vi "Mindsensors RTC-NX Config.vi"(10 "Node Data":T1, 11 "NXT":T2) -> ()   [LabVIEW 2010]
uses:
  <vilib>/NXT/Subs/LVHSConnector.ctl
  Datatypes/Node.ctl
  UI Controls/PlugInControls/Pluginbackground.ctl
  <vilib>/Utility/miscctls.llb/LVPointTypeDef.ctl
  ConvertNodeAddrSensor.vi
panel:
  out "Date":string
  out "Time":string
  in  "Clock Reading:":string
  out "?":u8 format="%x"
  out "?":dbl format="%#.2g"
  out "number":i8
  in  "Device Address":string
  in  "NXT Port":string
  in  "Name":string
  out "Headline":string="Type (auto populated)"
  in  "Sensor Parameters":string
  in  "Instance Specific Data":cluster{"Example Data":dbl}
  in  "Reset":bool
  in  "Save":bool
  in  "Stop":bool
  out "Background":T3=TRUE
  # "<- No controls below this line"
  # "Common controls such as Buttons, Rings, Sliders, Graphs, Decorations, etc can be found in the <labview>\\Targets\\NI\\NXT\\NXT Toolkit\\Schematic Editor\\UI Controls\\Plugin Controls\\ folder. Use these controls when possible to ensure a consistent look and feel with LabVIEW Education Edition."
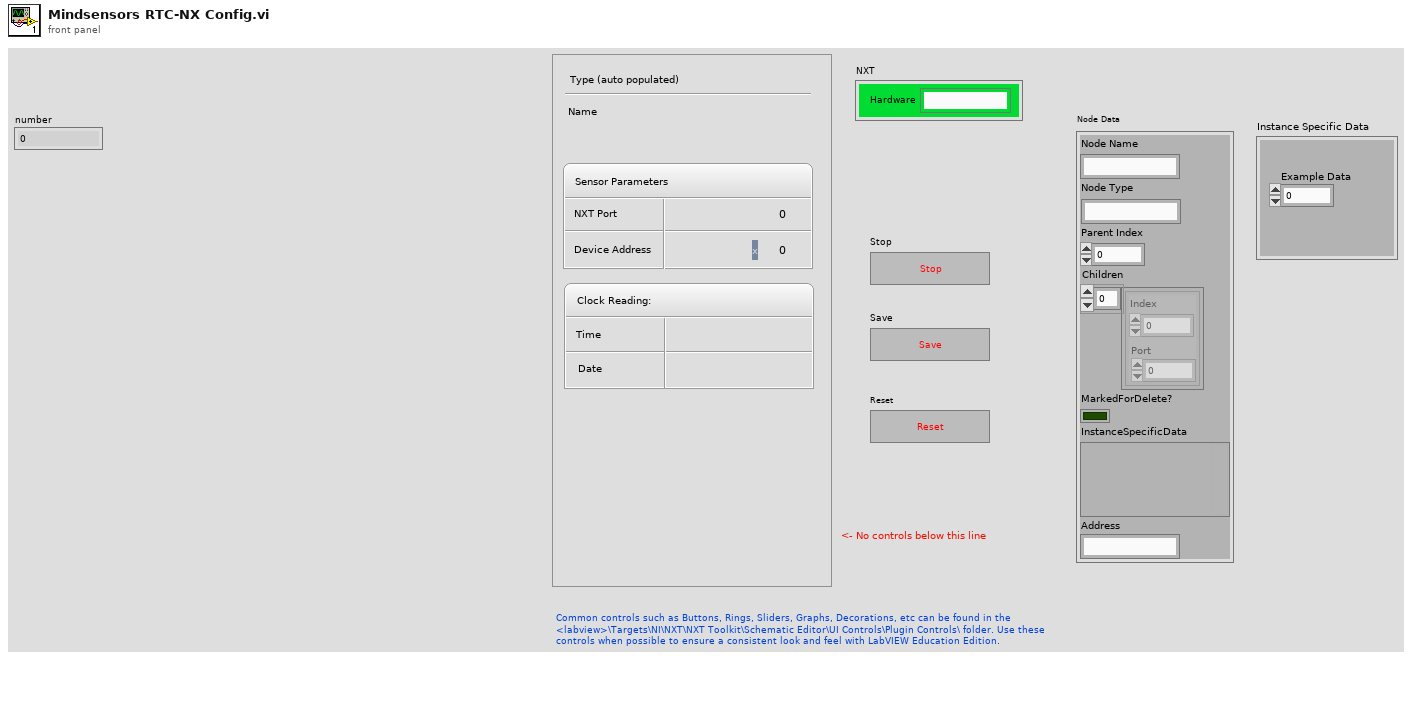
[diagram p1: front panel]
types:
  T1 = typedef "Node.ctl" = cluster{"Node Name":string, "Node Type":string, "Parent Index":i16, "Children":cluster{"Index":u16, "Port":u16}[], "MarkedForDelete?":bool, "InstanceSpecificData":variant, "Address":string}
  T2 = typedef "LVHSConnector.ctl" = cluster{"Hardware":string, "Flattened String":string}
  T3 = typedef "Pluginbackground.ctl" = bool
  T4 = typedef "LVPointTypeDef.ctl" = cluster{"Horizontal":i16, "Vertical":i16}
  T5 = enum8{"Enabled", "Disabled", "Disabled and Grayed Out"}
  T6 = typedef "NXT_InputPort.ctl" = u8
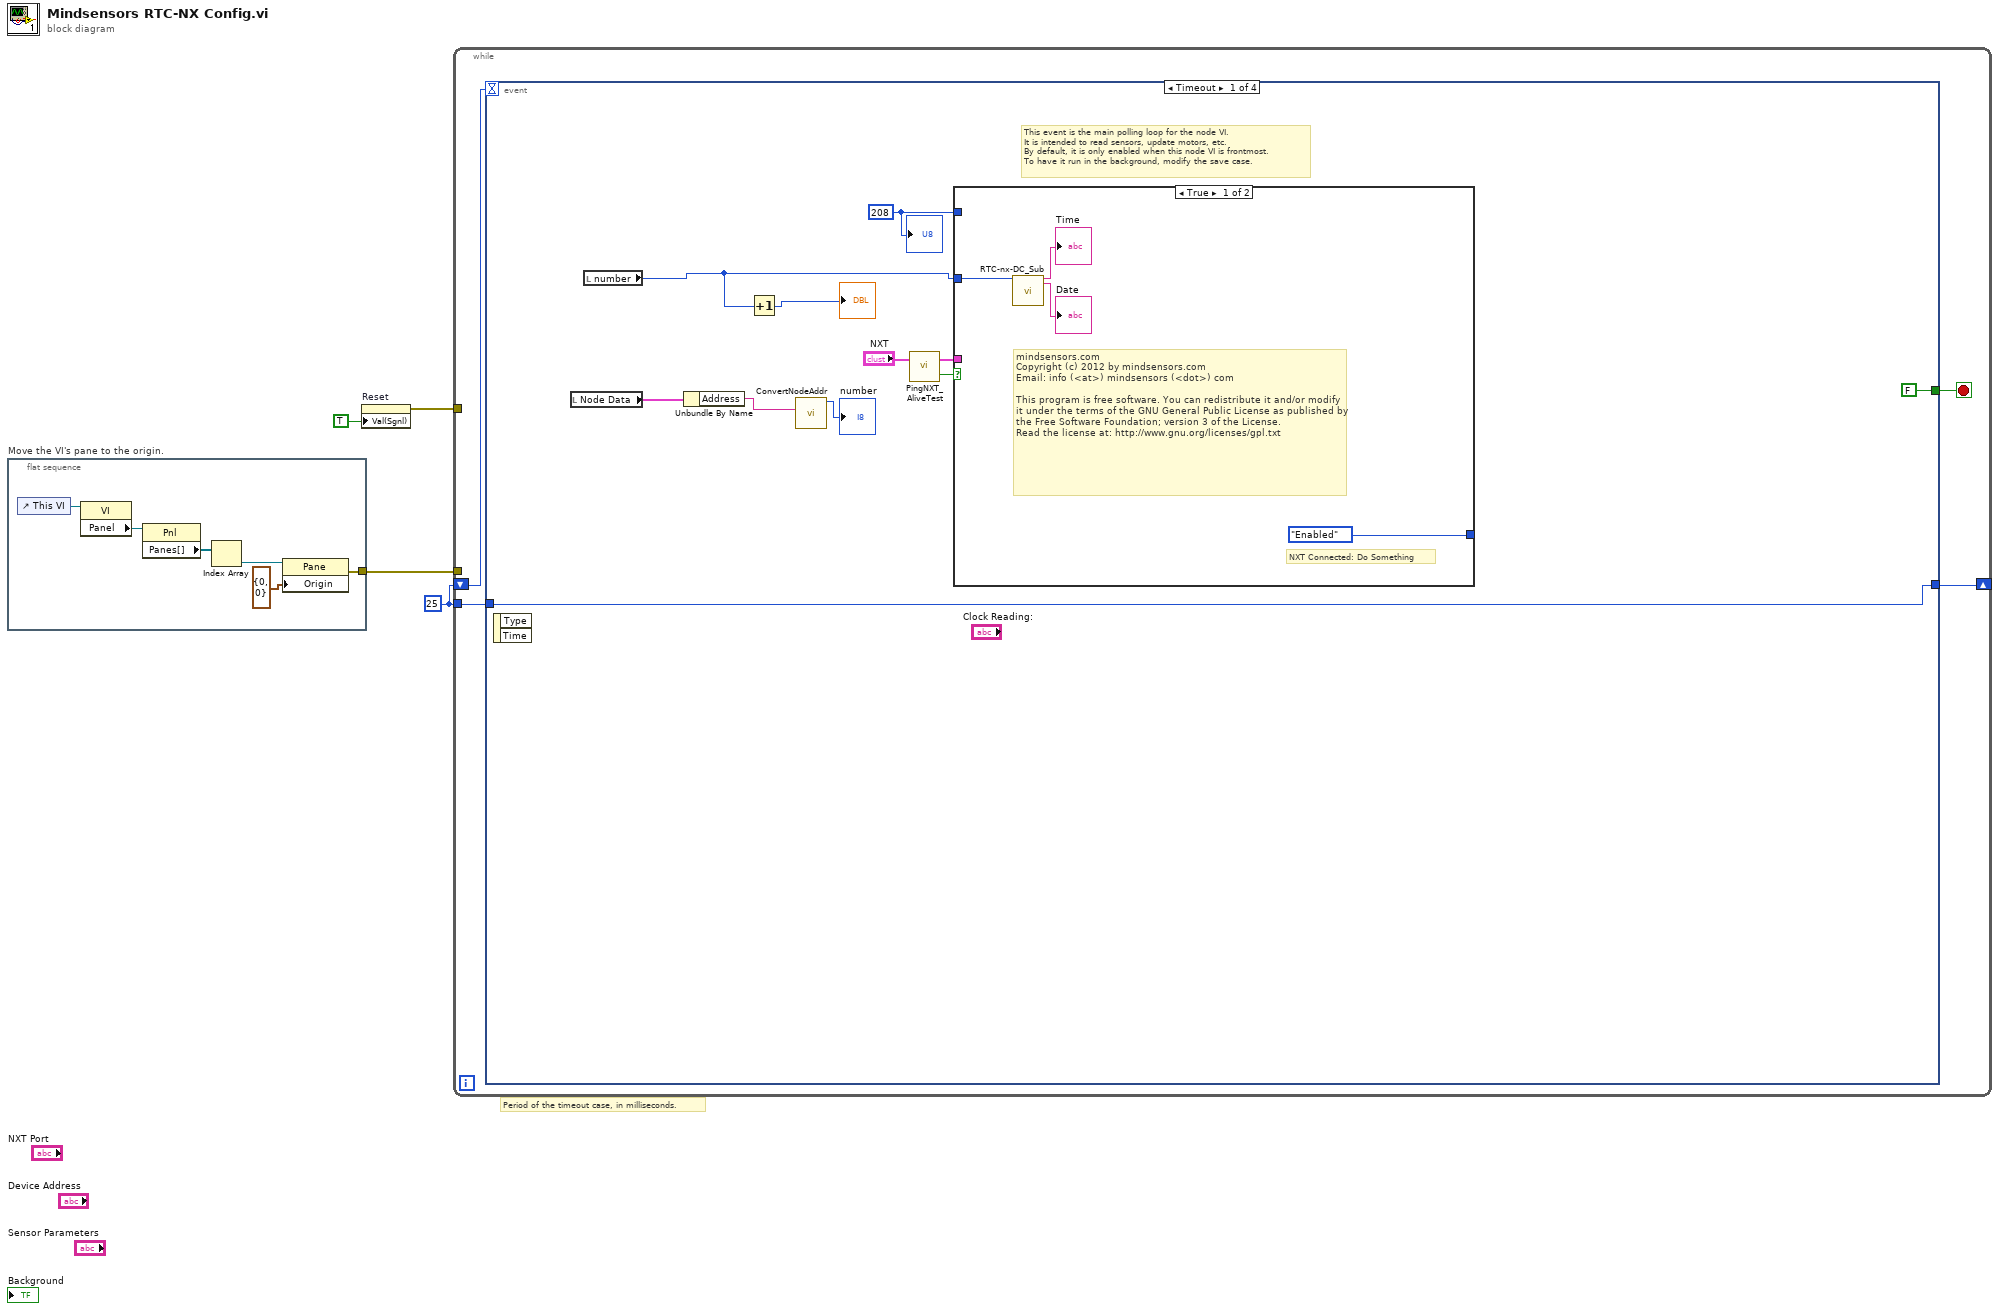
[diagram p0: block diagram]
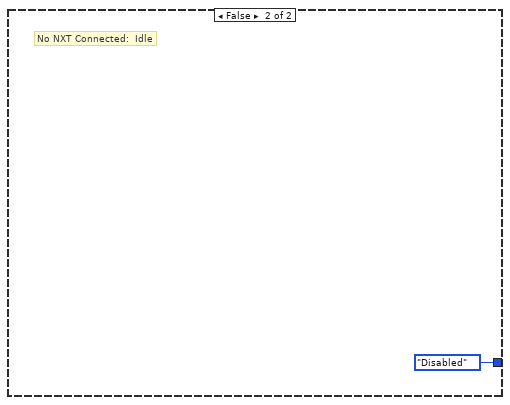
[diagram p2: hidden frame]
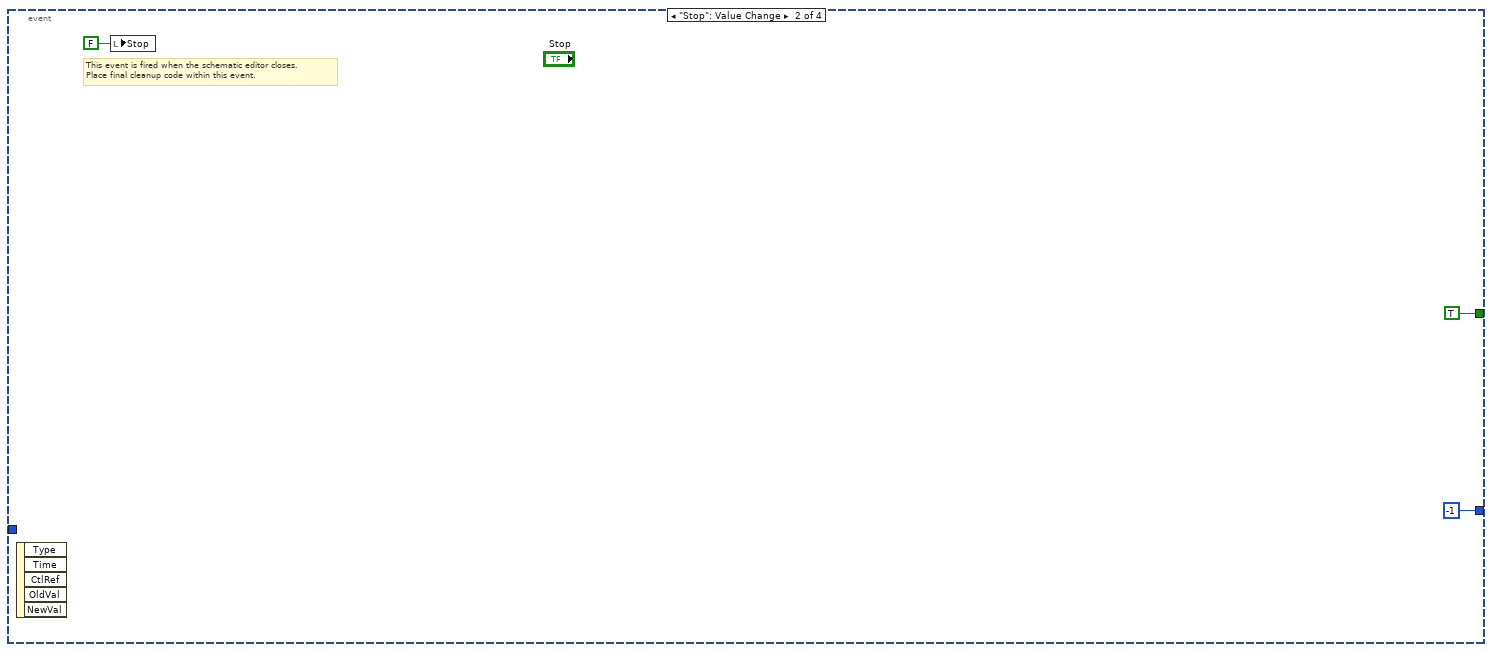
[diagram p3: hidden frame]
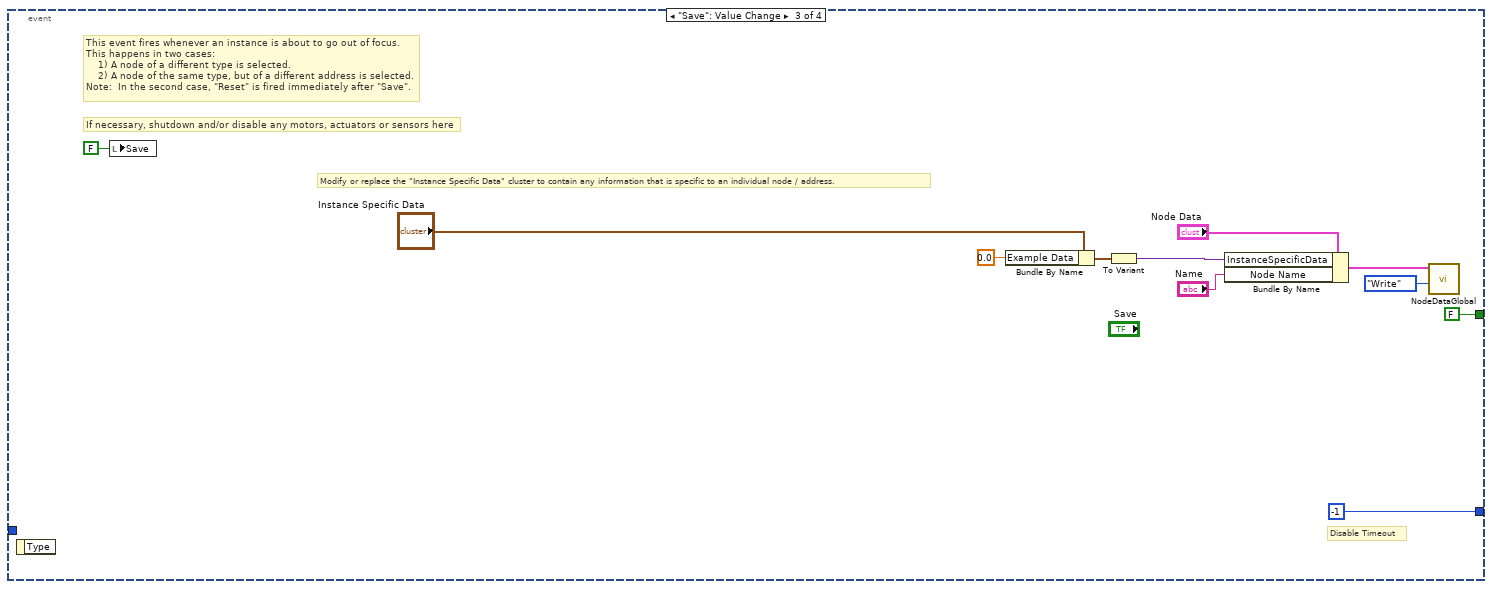
[diagram p4: hidden frame]
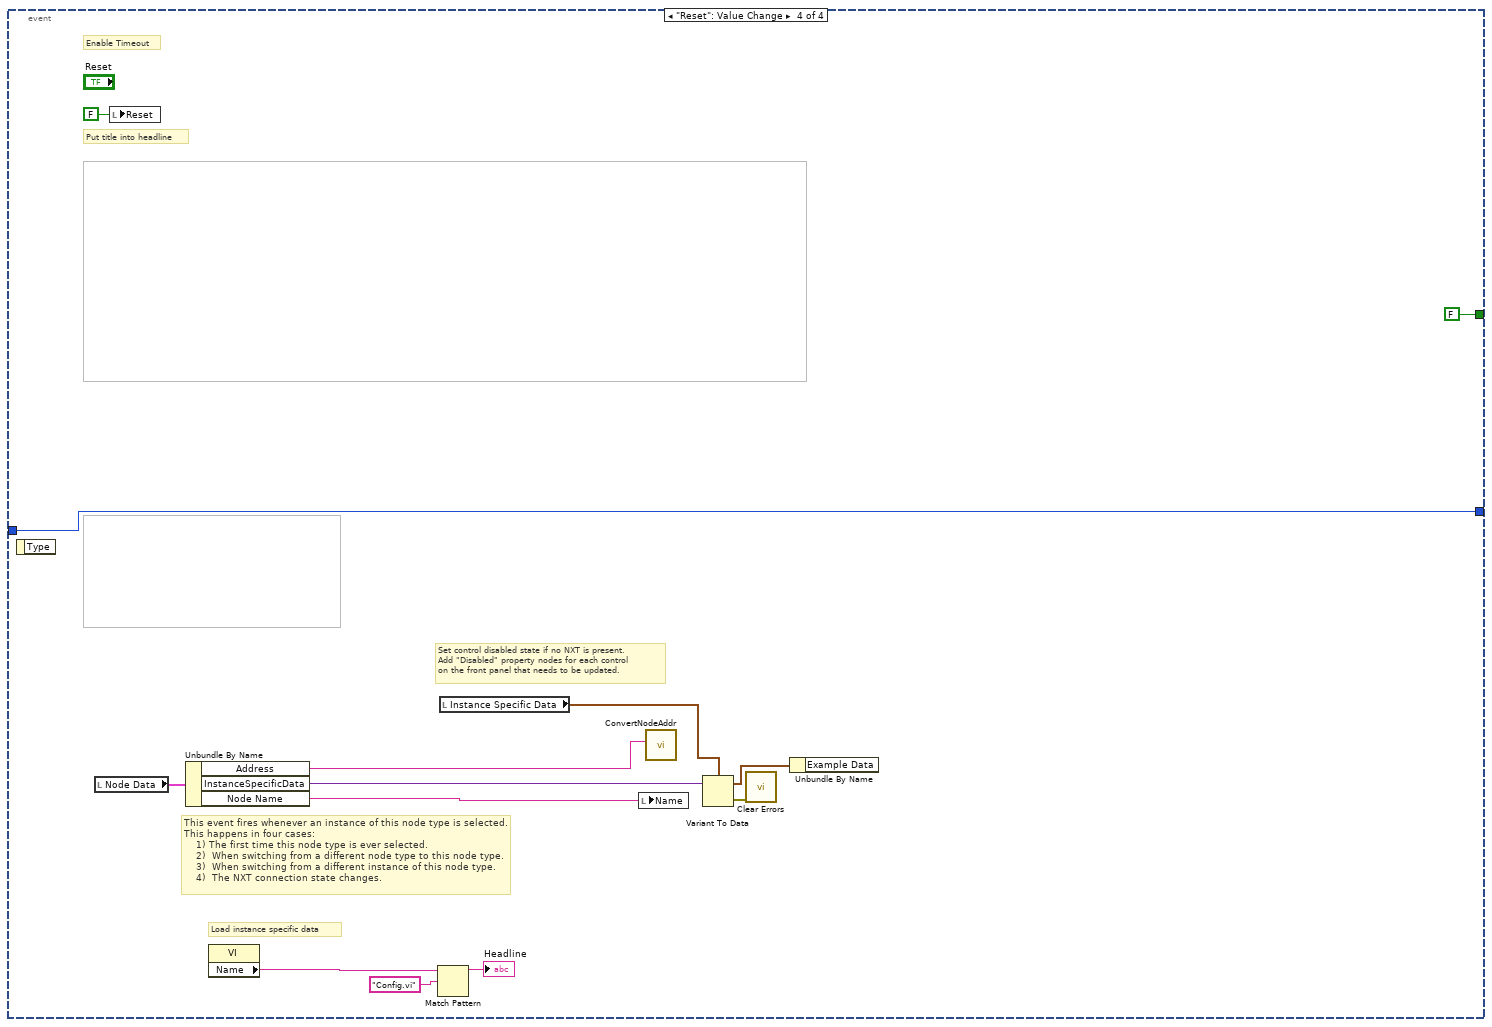
[diagram p5: hidden frame]
diagram:
  w2 = 25
  # "Period of the timeout case, in milliseconds."
  n1 = flat-sequence "Move the VI's pane to the origin." {
    tunnel: [w5] -> w1
    frame #0 {
      n2 = control-ref of="This VI"() -> (w6:refnum<vi>)
      n3 = property class="VI"(reference=w6) -> ("Panel"=w7:refnum<vi>)  [unwired: 1 in, 2 out]
      n4 = property class="Pnl"(reference=w7) -> ("Panes[]"=w8:refnum<vi>[])  [unwired: 1 in, 2 out]
      n5 = Index Array(array=w8) -> (element=w9:refnum<vi>)  [unwired: 1 in]
      n6 = property class="Pane"(reference=w9, "Origin"=T4 {"Horizontal"=0, "Vertical"=0}) -> (error out=w5:errorcluster)  [unwired: 1 in, 1 out]
    }
  }
  n7 = property on="Reset" class="Bool (strict)"("Val(Sgnl)"=TRUE ("Value (Signaling)")) -> (error out=w3:errorcluster)  [unwired: 2 in, 1 out]
  n8 = while {
    tunnel: w3 -> [_]
    shift-right: [w12] -> _
    shift-left: w2 -> [w13]
    tunnel: w2 -> [w11]
    tunnel: w1 -> [_]
    stop <- w14 stop-if-true
    n9 = event shown="[0] Timeout" {
      selector: _ -> [_ _ _ _]
      dyn-events: _ -> [_ _ _ _]
      timeout: w13 -> [_ _ _ _]
      tunnel: [FALSE TRUE FALSE FALSE] -> w14
      tunnel: [w24 -1 -1 w53] -> w12
      tunnel: w11 -> [w24 _ _ w53]
      event Timeout {
        w19 = 208 ("Registry Address")
        # "This event is the main polling loop for the node VI.\nIt is intended to read sensors, update motors, etc.\nBy default, it is only enabled when this node VI is frontmost.\nTo have it run in the background, modify the save case."
        n10 = event-data() -> ()  [unwired: 1 in, 2 out]
        n11 = local read "Node Data"() -> (w22:T1)
        n12 = local read "number"() -> (w16:i8)
        n13 = Unbundle By Name(w22) -> ("Address"=w18:string)
        n14 = Increment(x=w16) -> (x+1=→"?":i8)
        n15 = call-poly "ConvertNodeAddr.vi"("Sensor Port"=w18) -> ("NXT Port"=→"number":T6)  [unwired: 6 in, 4 out]
        n16 = call <vilib>:"PingNXT_AliveTest.vi"("NXT"="NXT") -> ("connected?"=w21:bool, "NXT"=w20:T2)  [unwired: 1 in]
        n17 = case shown="True" w21 {
          tunnel: [T5."Enabled" ("Disabled") T5."Disabled" ("Disabled")] -> _
          tunnel: w20 -> [_ _]
          tunnel: w16 -> [w28 _]
          tunnel: w19 -> [_ _]
          frame True {
            # "mindsensors.com\nCopyright (c) 2012 by mindsensors.com\nEmail: info (<at>) mindsensors (<dot>) com\n\nThis program is free software. You can redistribute it and/or modify\nit under the terms of the GNU General Public License as published by\nthe Free Software Foundation; version 3 of the License.\nRead the license at: http://www.gnu.org/licenses/gpl.txt"
            # "NXT Connected: Do Something"
            n18 = call <vilib>:"RTC-nx-DC_Sub.vi"("Input Port (Port 1)"=w28) -> ("time string"=→"Time":string, "date string"=→"Date":string)  [unwired: 10 in, 7 out]
          }
          frame False {
            # "No NXT Connected:  Idle"
          }
        }
        "?" <- w19
      }
      event "Stop": Value Change {
        # "This event is fired when the schematic editor closes.\nPlace final cleanup code within this event."
        n19 = event-data() -> ()  [unwired: 1 in, 5 out]
        n20 = local write "Stop"(FALSE ("stop")) -> ()
      }
      event "Save": Value Change {
        # "If necessary, shutdown and/or disable any motors, actuators or sensors here"
        # "Modify or replace the \"Instance Specific Data\" cluster to contain any information that is specific to an individual node / address."
        # "Disable Timeout"
        # "This event fires whenever an instance is about to go out of focus.\nThis happens in two cases:\n    1) A node of a different type is selected.\n    2) A node of the same type, but of a different address is selected.\nNote:  In the second case, \"Reset\" is fired immediately after \"Save\"."
        n21 = event-data() -> ()  [unwired: 1 in, 1 out]
        n22 = local write "Save"(FALSE ("stop")) -> ()
        n23 = Bundle By Name(cluster="Instance Specific Data", "Example Data"=0.0) -> (w35:cluster{"Example Data":dbl})
        n24 = To Variant(anything=w35) -> (Variant=w42:variant)
        n25 = Bundle By Name(cluster="Node Data", "InstanceSpecificData"=w42, "Node Name"="Name") -> (w41:T1)
        n26 = call "NodeDataGlobal.vi"("Action"=enum16{"Read", "Write"}."Write", "Node Data In"=w41) -> ()  [unwired: 8 in, 2 out]
      }
      event "Reset": Value Change {
        # "Set control disabled state if no NXT is present.\nAdd \"Disabled\" property nodes for each control\non the front panel that needs to be updated."
        # "Load instance specific data"
        # "Enable Timeout"
        # "This event fires whenever an instance of this node type is selected.\nThis happens in four cases:\n    1) The first time this node type is ever selected.\n    2)  When switching from a different node type to this node type.\n    3)  When switching from a different instance of this node type. \n    4)  The NXT connection state changes."
        # "Put title into headline"
        n27 = event-data() -> ()  [unwired: 1 in, 1 out]
        n28 = local read "Node Data"() -> (w54:T1)
        n29 = local write "Reset"(FALSE ("Reset")) -> ()
        n30 = Unbundle By Name(w54) -> ("Address"=w45:string, "InstanceSpecificData"=w55:variant, "Node Name"=w47:string)
        n31 = property class="VI"() -> ("Name"=w49:string)  [unwired: 2 in, 2 out]
        n32 = Match Pattern(string=w49, regular expression="Config.vi") -> (before substring=→"Headline":string)  [unwired: 1 in, 3 out]
        n33 = local read "Instance Specific Data"() -> (w52:cluster{"Example Data":dbl})
        n34 = local write "Name"(w47) -> ()
        n35 = call-poly "ConvertNodeAddr.vi"("Sensor Port"=w45) -> ()  [unwired: 6 in, 5 out]
        n36 = Variant To Data(Variant=w55, type=w52) -> (error out=w51:errorcluster, data=w46:cluster{"Example Data":dbl})  [unwired: 1 in]
        n37 = call <vilib>:"Clear Errors.vi"("error in (no error)"=w51) -> ()  [unwired: 6 in, 1 out]
        n38 = Unbundle By Name(w46) -> ()  [unwired: 1 out]
      }
    }
  }
